vi "LJM logger process scaling equation error.vi"(3 "Error In":errorcluster, 4 "Scaling Equation Index":i32, 5 "Bad Formula":string) -> (0 "Error Out":errorcluster)   [LabVIEW 2026]
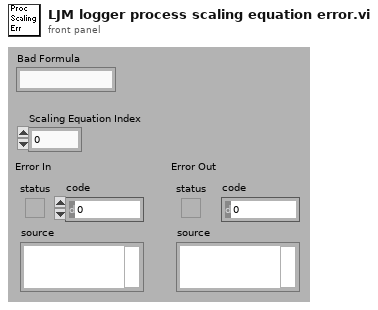
[diagram p1: front panel]
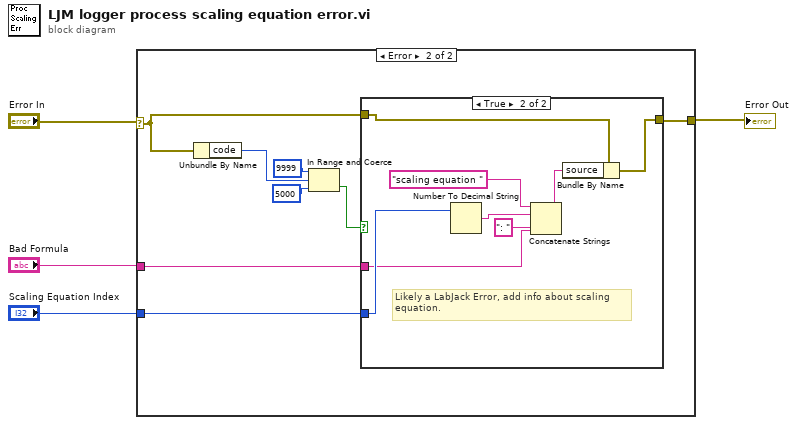
[diagram p0: block diagram]
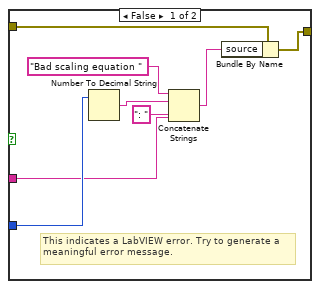
[diagram p3: hidden frame]
diagram:
  n1 = case shown="Error" "Error In" {
    selector: "Error In" -> [w5 w8]
    tunnel: "Bad Formula" -> [_ w13]
    tunnel: [w5 w12] -> w3
    tunnel: "Scaling Equation Index" -> [_ w6]
    frame No Error {
    }
    frame Error {
      n2 = Unbundle By Name(w8) -> ("code"=w9:i32)
      n3 = In Range and Coerce(upper limit=9999, x=w9, lower limit=5000) -> (In Range?=w7:bool)  [unwired: 1 out]
      n4 = case shown="True" w7 {
        tunnel: w13 -> [w15 w25]
        tunnel: w8 -> [w20 w23]
        tunnel: [w18 w22] -> w12
        tunnel: w6 -> [w16 w26]
        frame False {
          # "This indicates a LabVIEW error. Try to generate a\nmeaningful error message."
          n5 = Number To Decimal String(number=w16) -> (decimal integer string=w17:string)  [unwired: 1 in]
          n6 = Concatenate Strings("Bad scaling equation ", w17, ": " ("string"), w15) -> (w19:string)
          n7 = Bundle By Name(cluster=w20, "source"=w19) -> (w18:errorcluster)
        }
        frame True {
          # "Likely a LabJack Error, add info about scaling\nequation."
          n8 = Number To Decimal String(number=w26) -> (decimal integer string=w28:string)  [unwired: 1 in]
          n9 = Concatenate Strings("scaling equation ", w28, ": " ("string"), w25) -> (w24:string)
          n10 = Bundle By Name(cluster=w23, "source"=w24) -> (w22:errorcluster)
        }
      }
    }
  }
  "Error Out" <- w3
